vi "Write subindex.vi"(8 "error in":errorcluster, 10 "subindex":i32, 11 "EthernetIP Channel in":refnum<class "EthernetIP Channel.lvclass">) -> (0 "error out":errorcluster, 3 "EthernetIP Channel out":refnum<class "EthernetIP Channel.lvclass">)   [LabVIEW 2013, in "EthernetIP Channel.lvclass"]
uses:
  EthernetIP Channel.lvclass
  EthernetIP Channel.lvclass/EthernetIP Channel.ctl
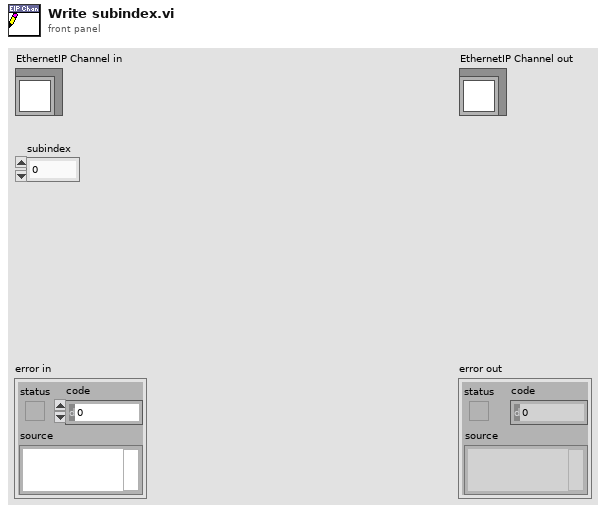
[diagram p1: front panel]
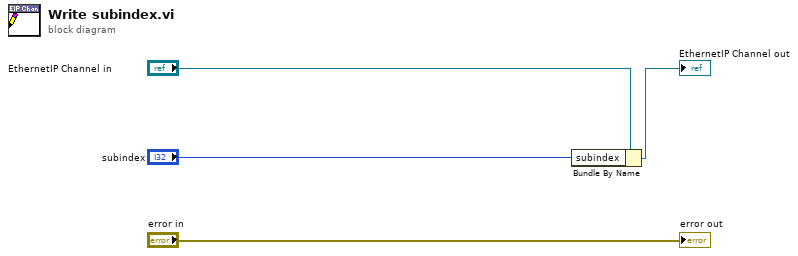
[diagram p0: block diagram]
diagram:
  n1 = Bundle By Name(cluster="EthernetIP Channel in", "subindex"="subindex") -> (→"EthernetIP Channel out":refnum<class "EthernetIP Channel.lvclass">)
  "error out" <- "error in"
